vi "Set Address.vi"(6 "chip select  (1st chip)":enum16{"1st chip", "2nd chip"}(ring), 8 "error in (no error)":errorcluster, 9 "address":u8 format="%.0x", 10 "address type (DDRAM)":enum16{"DDRAM", "CGRAM"}(ring), 11 "HD44780 in":refnum<class "HD44780.lvclass">) -> (0 "error out":errorcluster, 3 "HD44780 out":refnum<class "HD44780.lvclass">)   [LabVIEW 2017, in "HD44780.lvclass"]
uses:
  HD44780.lvclass
  HD44780.lvclass/HD44780.ctl
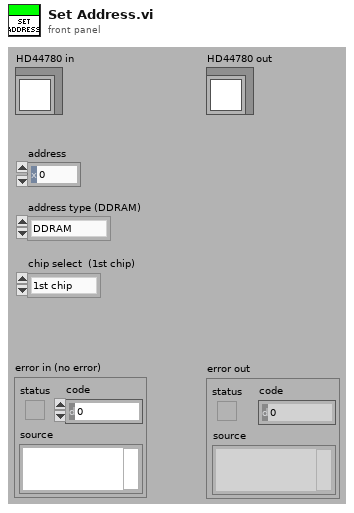
[diagram p1: front panel]
types:
  T1 = typedef "HD44780 Common.lvlib/cluster of class private data.ctl" = cluster{"FPGA VI Reference":refnum<k20>, "device index":i8, "screen size":T2, "font size":T3, "auto wrap":bool, "alignment":T4, "number of line":T5, "shift 0":i8, "entry mode 0":T6, "shift 1":i8, "entry mode 1":T6}
  T2 = typedef "HD44780 Common.lvlib/screen size.ctl" = enum8{"8x1", "8x2", "12x4", "16x1", "16x2", "16x4", "20x1", "20x2", "20x4", "24x1", "24x2", "40x2", "40x4"}
  T3 = typedef "HD44780 Common.lvlib/font size.ctl" = enum8{"5x8", "5x10"}
  T4 = typedef "HD44780 Common.lvlib/alignment.ctl" = enum16{"None", "Left", "Center", "Right"}
  T5 = typedef "HD44780 Common.lvlib/line number.ctl" = enum8{"1 line", "2 lines"}
  T6 = typedef "HD44780 Common.lvlib/entry mode.ctl" = enum8{"increment & no shift", "increment & shift", "decrement & no shift", "decrement & shift"}
  T7 = cluster{"FPGA VI Reference":refnum<k20>, "device index":i8, "screen size":enum8{"8x1", "8x2", "12x4", "16x1", "16x2", "16x4", "20x1", "20x2", "20x4", "24x1", "24x2", "40x2", "40x4"}, "font size":enum8{"5x8", "5x10"}, "auto wrap":bool, "alignment":enum16{"None", "Left", "Center", "Right"}, "number of line":enum8{"1 line", "2 lines"}, "shift 0":i8, "entry mode 0":enum8{"increment & no shift", "increment & shift", "decrement & no shift", "decrement & shift"}, "shift 1":i8, "entry mode 1":enum8{"increment & no shift", "increment & shift", "decrement & no shift", "decrement & shift"}}
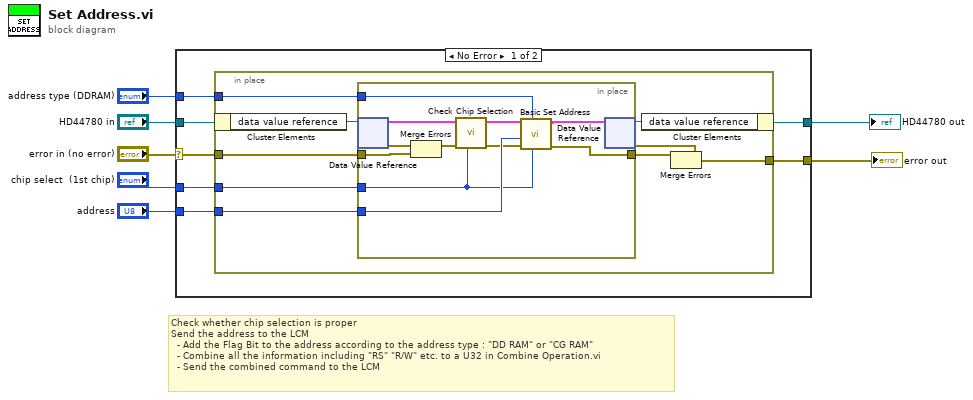
[diagram p0: block diagram]
diagram:
  # "Check whether chip selection is proper\nSend the address to the LCM\n  - Add the Flag Bit to the address according to the address type : \"DD RAM\" or \"CG RAM\" \n  - Combine all the information including \"RS\" \"R/W\" etc. to a U32 in Combine Operation.vi \n  - Send the combined command to the LCM"
  n1 = case shown="No Error" "error in (no error)" {
    selector: "error in (no error)" -> [w13 w36]
    tunnel: [w14 w36] -> w7
    tunnel: "HD44780 in" -> [w9 w35]
    tunnel: "address type (DDRAM)" -> [w12 _]
    tunnel: "address" -> [w11 _]
    tunnel: "chip select  (1st chip)" -> [w10 _]
    tunnel: [w8 w35] -> w1
    frame No Error {
      n2 = in-place {
        in-place-border: [w21] -> w14
        in-place-border: w13 -> [w20]
        in-place-border: w12 -> [w19]
        in-place-border: w11 -> [w18]
        in-place-border: w10 -> [w17]
        n3 = in-place-cluster #1(w9) -> ("data value reference"=w16:refnum<data-value>)
        n4 = in-place {
          in-place-border: [w34] -> w22
          in-place-border: w20 -> [w31]
          in-place-border: w19 -> [w30]
          in-place-border: w18 -> [w29]
          in-place-border: w17 -> [w24]
          n5 = in-place-dvr #2(w16) -> (w28:T1, w32:errorcluster)
          n6 = Merge Errors(w32, w31) -> (w25:errorcluster)
          n7 = call "Check Chip Selection.vi"("chip select"=w24, "error in (no error)"=w25, "cluster of private data in"=w28) -> ("error out"=w26:errorcluster, "cluster of private data out"=w27:T7)  [unwired: 7 in]
          n8 = call "Basic Set Address.vi"("chip select  (1st chip)"=w24, "address type (DDRAM)"=w30, "error in (no error)"=w26, "address (0, 0)"=w29, "cluster of private data in"=w27) -> ("error out"=w34:errorcluster, "cluster of private data out"=w33:T7)  [unwired: 5 in]
          n9 = in-place-dvr #2(w33) -> (w15:refnum<data-value>, w23:errorcluster)
        }
        n10 = in-place-cluster #1("data value reference"=w15) -> (w8:refnum<class "HD44780.lvclass">)
        n11 = Merge Errors(w23, w22) -> (w21:errorcluster)
      }
    }
    frame Error {
    }
  }
  "error out" <- w7
  "HD44780 out" <- w1
